vi "send and receive.vi"(10 "write to laser":string, 11 "VISA resource name":refnum<visa-resource-name>) -> (2 "read from laser":string, 3 "VISA resource name out":refnum<visa-resource-name>)   [LabVIEW 8.6]
panel:
  # "This VI sends and receives commands to the laser.  This VI is used as the lower-level communication VI for the rest of the VIs included here."
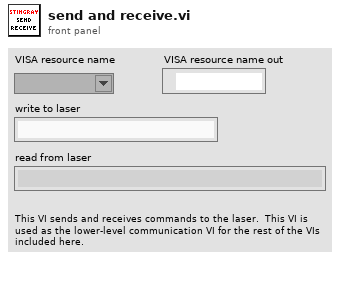
[diagram p1: front panel]
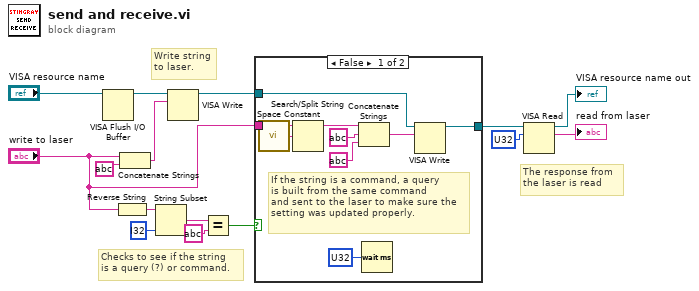
[diagram p0: block diagram]
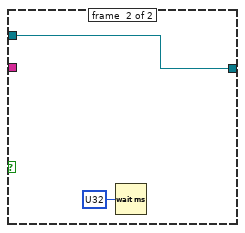
[diagram p2: hidden frame]
diagram:
  # "The response from\nthe laser is read"
  # "Checks to see if the string\nis a query (?) or command."
  # "Write string\nto laser."
  n1 = VISA Flush I/O Buffer(VISA resource name="VISA resource name") -> (VISA resource name out=w5:refnum<visa-resource-name>)  [unwired: 2 in, 1 out]
  n2 = Reverse String(1:"write to laser") -> (0:w12:string)
  n3 = Concatenate Strings("write to laser", string ?) -> (w14:string)
  n4 = String Subset(string=w12, length (rest)=i32 ? ("length (rest)")) -> (substring=w10:string)  [unwired: 1 in]
  n5 = VISA Write(VISA resource name=w5, write buffer=w14) -> (VISA resource name out=w13:refnum<visa-resource-name>)  [unwired: 1 in, 2 out]
  n6 = Equal?(x=w10, y=string ?) -> (x = y?=w8:bool)
  n7 = case shown="False" w8 {
    tunnel: w13 -> [w20 w26]
    tunnel: [w19 w26] -> w7
    tunnel: "write to laser" -> [w16 _]
    frame #0 {
      # "If the string is a command, a query\nis built from the same command\nand sent to the laser to make sure the\nsetting was updated properly."
      n8 = call <vilib>:"Space Constant.vi"() -> ("String"=w24:string)
      n9 = Search/Split String(string=w16, search string/char (-)=w24) -> (substring before match=w23:string)  [unwired: 1 in, 2 out]
      n10 = Concatenate Strings(w23, string ? ("string"), string ?) -> (w21:string)
      n11 = Wait (ms)(milliseconds to wait=u32 ?) -> ()  [unwired: 1 out]
      n12 = VISA Write(VISA resource name=w20, write buffer=w21) -> (VISA resource name out=w19:refnum<visa-resource-name>)  [unwired: 1 in, 2 out]
    }
    frame #1 {
      n13 = Wait (ms)(milliseconds to wait=u32 ?) -> ()  [unwired: 1 out]
    }
  }
  n14 = VISA Read(VISA resource name=w7, byte count=u32 ?) -> (VISA resource name out=→"VISA resource name out":refnum<visa-resource-name>, read buffer=→"read from laser":string)  [unwired: 1 in, 2 out]
